vi "About Window.vi"() -> ()   [LabVIEW 2018]
panel:
  in  "Cancel Button":bool
  out "String":string
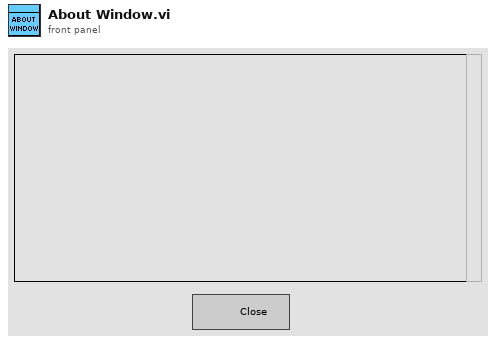
[diagram p1: front panel]
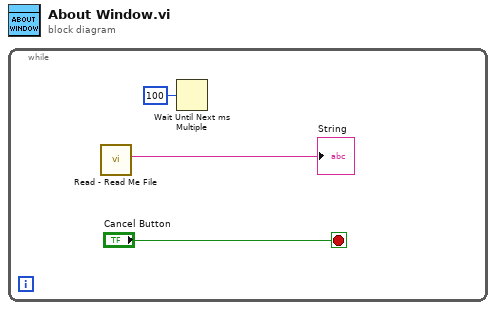
[diagram p0: block diagram]
diagram:
  n1 = while {
    stop <- "Cancel Button" stop-if-true
    n2 = call "Read - Read Me File.vi"() -> ("full text"=→"String":string)  [unwired: 10 in, 1 out]
    n3 = Wait Until Next ms Multiple(millisecond multiple=u32 100) -> ()  [unwired: 1 out]
  }
